vi "Do.vi"(8 "error in (no error)":errorcluster, 10 "Actor in":refnum<class "Actor.lvclass">, 11 "EMS Setpoint Msg":refnum<class "EMS Setpoint Status Msg.lvclass">) -> (0 "error out":errorcluster, 2 "Actor out":refnum<class "Actor.lvclass">)   [LabVIEW 2015, in "Master Controller Core.lvlib" / "EMS Setpoint Status Msg.lvclass"]
uses:
  EMS Setpoint Status Msg.lvclass
  <vilib>/ActorFramework/Actor/Actor.lvclass
  Master Controller/Master Controller.lvclass
  SCADA Core/SCADA Abstract Messages/IED Setpoint Status Msg/IED Setpoint Status Msg.lvclass/IED Setpoint Status Msg.ctl
  SCADA Core/SCADA Abstract Messages/IED Setpoint Status Msg/IED Setpoint Status Msg.lvclass
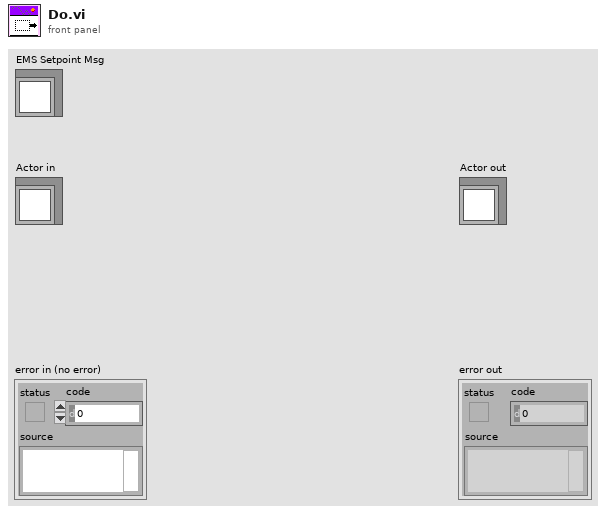
[diagram p1: front panel]
types:
  T1 = typedef "SCADA Core.lvlib/IED Setpoint Status Msg.lvclass/IED Setpoint Status.ctl" = enum16{"Success", "Failure", "Multiple Success", "Multiple Failure"}
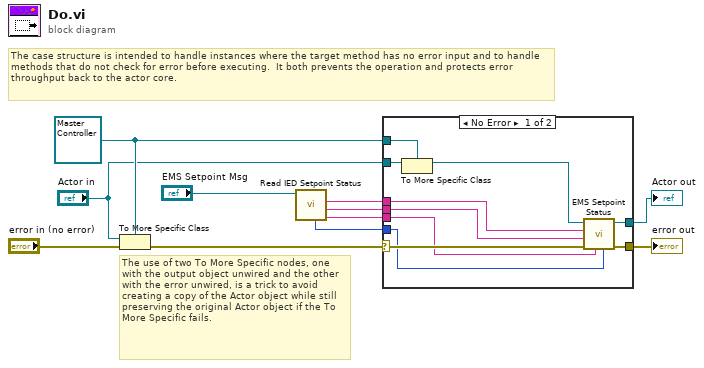
[diagram p0: block diagram]
diagram:
  w11 = refnum<class "Master Controller.lvclass"> refnum ("Actor in")
  # "The use of two To More Specific nodes, one with the output object unwired and the other with the error unwired, is a trick to avoid creating a copy of the Actor object while still preserving the original Actor object if the To More Specific fails."
  # "The case structure is intended to handle instances where the target method has no error input and to handle methods that do not check for error before executing.  It both prevents the operation and protects error throughput back to the actor core."
  n1 = To More Specific Class(target class=w11, reference="Actor in", error in="error in (no error)") -> (error out=w7:errorcluster)  [unwired: 1 out]
  n2 = call "Read IED Setpoint Status.vi"("IED Setpoint Status Msg in"="EMS Setpoint Msg") -> ("Error String"=w2:string, "Variable Name"=w3:string, "IED Name"=w4:string, "Status"=w1:T1)  [unwired: 6 in, 1 out]
  n3 = case shown="No Error" w7 {
    selector: w7 -> [w17 w23]
    tunnel: [w16 w23] -> w8
    tunnel: [w19 w22] -> w9
    tunnel: "Actor in" -> [w21 w22]
    tunnel: w11 -> [w20 _]
    tunnel: w4 -> [w15 _]
    tunnel: w3 -> [w14 _]
    tunnel: w2 -> [w13 _]
    tunnel: w1 -> [w12 _]
    frame No Error {
      n4 = To More Specific Class(target class=w20, reference=w21) -> (specific class reference=w18:refnum<class "Master Controller.lvclass">)  [unwired: 1 in, 1 out]
      n5 = call-dynamic "EMS Setpoint Status.vi"("Status"=w12, "Error String"=w13, "error in (no error)"=w17, "Variable Name"=w14, "IED Name"=w15, "Master Controller in"=w18) -> ("error out"=w16:errorcluster, "Master Controller out"=w19:refnum<class "Master Controller.lvclass">)  [unwired: 4 in]
    }
    frame Error {
      # "If type check fails, pass the original object out again."
    }
  }
  "error out" <- w8
  "Actor out" <- w9
